vi "WriteToDb.vi"(0 "reference in":refnum<class "AO.lvclass">, 11 "error in (no error)":errorcluster) -> (4 "reference out":refnum<class "AO.lvclass">, 15 "error out":errorcluster)   [LabVIEW 2019, in "AO.lvclass"]
uses:
  AO.lvclass
  D:/GIT H4000/H4000/src/Proccess_class/Proccess.lvclass
  Proccess_class/Proccess.lvclass/Proccess.ctl
  AO.lvclass/AO.ctl
  Logger_class/SignalData.ctl
  Logger_class/Logger.lvclass/Logger.ctl
  Logger_class/Logger.lvclass
  Proccess_class/Proccess.lvclass
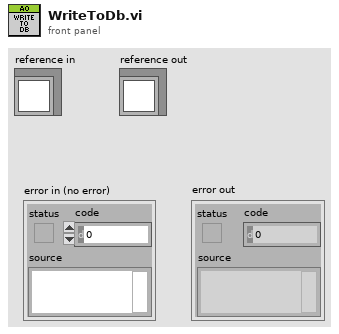
[diagram p1: front panel]
types:
  T1 = typedef "Logger.lvclass/SignalData.ctl" = cluster{"Value":dbl, "SignalTag":string, "ObjTag":string, "Desc":string, "Time Stamp":timestamp}
  T2 = typedef "Proccess.lvclass/TAGs.ctl" = cluster{"TAG":string, "PTAG":string, "DESC":string}
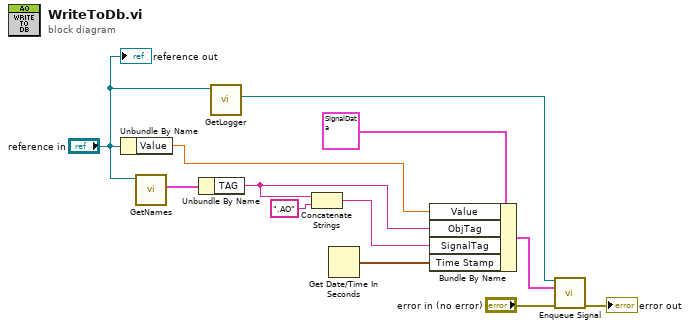
[diagram p0: block diagram]
diagram:
  n1 = Unbundle By Name("reference in") -> ("Value"=w7:dbl)
  n2 = call "GetNames.vi"("Proccess in"="reference in") -> ("Tags"=w4:T2)  [unwired: 10 in]
  n3 = Unbundle By Name(w4) -> ("TAG"=w1:string)
  n4 = call "GetLogger.vi"("Proccess in"="reference in") -> ("Logger"=w3:refnum<class "Logger.lvclass">)  [unwired: 10 in]
  n5 = Concatenate Strings(w1, ".AO" ("string")) -> (w10:string)
  n6 = Get Date/Time In Seconds() -> (seconds since 1Jan1904=w9:timestamp)
  n7 = Bundle By Name(cluster=T1 {"Value"=0.0, "SignalTag"="", "ObjTag"="", "Desc"="", "Time Stamp"=timestamp(0 s since 1904-01-01)} ("element"), "Value"=w7, "ObjTag"=w1, "SignalTag"=w10, "Time Stamp"=w9) -> (w5:T1)
  n8 = call "Enqueue Signal.vi"("reference in"=w3, "element"=w5, "error in (no error)"="error in (no error)") -> ("error out"=→"error out":errorcluster)  [unwired: 11 in, 1 out]
  "reference out" <- "reference in"
